vi "update_AnalysisList.vi"(8 "error in (no error)":errorcluster, 11 "Analysis List ref":refnum<vi>) -> (0 "error out":errorcluster)   [LabVIEW 2015]
uses:
  global_variables.vi
  Classes/AnalysisList/AnalysisList.lvclass
  Classes/AnalysisListItems/AnalysisListItems.lvclass
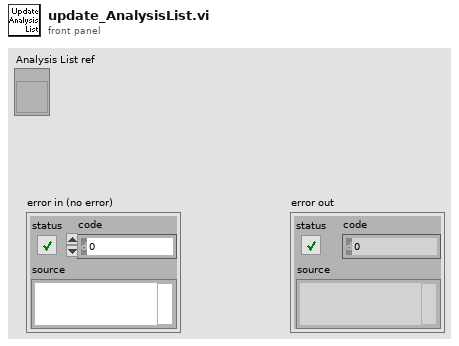
[diagram p1: front panel]
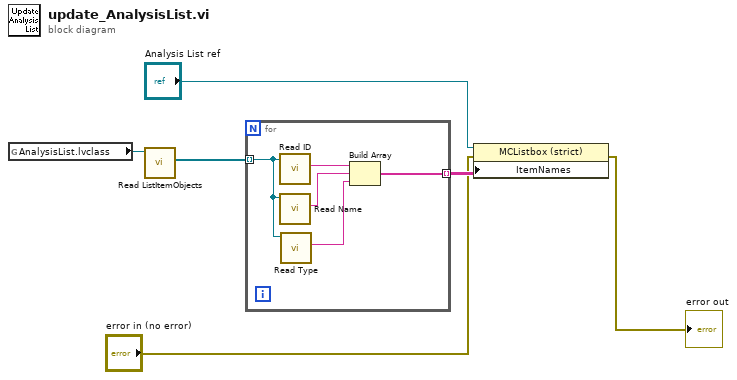
[diagram p0: block diagram]
diagram:
  n1 = global read "global_variables.vi" "AnalysisList.lvclass"() -> (w6:refnum<class "AnalysisList.lvclass">)
  n2 = call-dynamic "Read ListItemObjects.vi"("AnalysisList in"=w6) -> ("AnalysisObjects"=w5:refnum<class "AnalysisListItems.lvclass">[])  [unwired: 8 in, 2 out]
  n3 = for {
    tunnel: w5 -> [w11] mode=indexing
    tunnel: [w7] -> w4 mode=indexing
    n4 = call-dynamic "Read ID.vi"("AnalysisListItems in"=w11) -> ("ID"=w10:string)  [unwired: 8 in, 2 out]
    n5 = call-dynamic "Read Name.vi"("AnalysisListItems in"=w11) -> ("Name"=w9:string)  [unwired: 8 in, 2 out]
    n6 = call-dynamic "Read Type.vi"("AnalysisListItems in"=w11) -> ("Type"=w8:string)  [unwired: 8 in, 2 out]
    n7 = Build Array(w10, w9, w8) -> (w7:string[])
  }
  n8 = property class="MCListbox (strict)"(reference="Analysis List ref", error in="error in (no error)", "ItemNames"=w4) -> (error out=→"error out":errorcluster)  [unwired: 1 out]
